vi "MNK_TC_to_DSC.vi"(8 "error in (no error)":errorcluster, 9 "calibration string":string, 10 "description string":string, 11 "dbl":dbl[](array[numeric])) -> (0 "error out":errorcluster)   [LabVIEW 2016]
panel:
  in  "calibration string var":refnum<k21>="ni.var.psp://housesoftheholy/MNK_18T/MNK_TC_calibration"
  in  "description string var":refnum<k21>="ni.var.psp://housesoftheholy/MNK_18T/MNK_TC_description"
  in  "dbl var":refnum<k21>[](array[refnum])=["ni.var.psp://housesoftheholy/MNK_18T/MNK_TC_R0", "ni.var.psp://housesoftheholy/MNK_18T/MNK_TC_R1", "ni.var.psp://housesoftheholy/MNK_18T/MNK_TC_R2", "ni.var.psp://housesoftheholy/MNK_18T/MNK_TC_R3", "ni.var.psp://housesoftheholy/MNK_18T/MNK_TC_R4", "ni.var.psp://housesoftheholy/MNK_18T/MNK_TC_R5", "ni.var.psp://housesoftheholy/MNK_18T/MNK_TC_R6", "ni.var.psp://housesoftheholy/MNK_18T/MNK_TC_R7", "ni.var.psp://housesoftheholy/MNK_18T/MNK_TC_T0", "ni.var.psp://housesoftheholy/MNK_18T/MNK_TC_T1", "ni.var.psp://housesoftheholy/MNK_18T/MNK_TC_T2", "ni.var.psp://housesoftheholy/MNK_18T/MNK_TC_T3", "ni.var.psp://housesoftheholy/MNK_18T/MNK_TC_T4", "ni.var.psp://housesoftheholy/MNK_18T/MNK_TC_T5", "ni.var.psp://housesoftheholy/MNK_18T/MNK_TC_T6", "ni.var.psp://housesoftheholy/MNK_18T/MNK_TC_T7", "ni.var.psp://housesoftheholy/MNK_18T/MNK_TC_I0", "ni.var.psp://housesoftheholy/MNK_18T/MNK_TC_I1", "ni.var.psp://housesoftheholy/MNK_18T/MNK_TC_I2", "ni.var.psp://housesoftheholy/MNK_18T/MNK_TC_I3", "", "", "", "", ""]
  # "MNK TC to DSC"
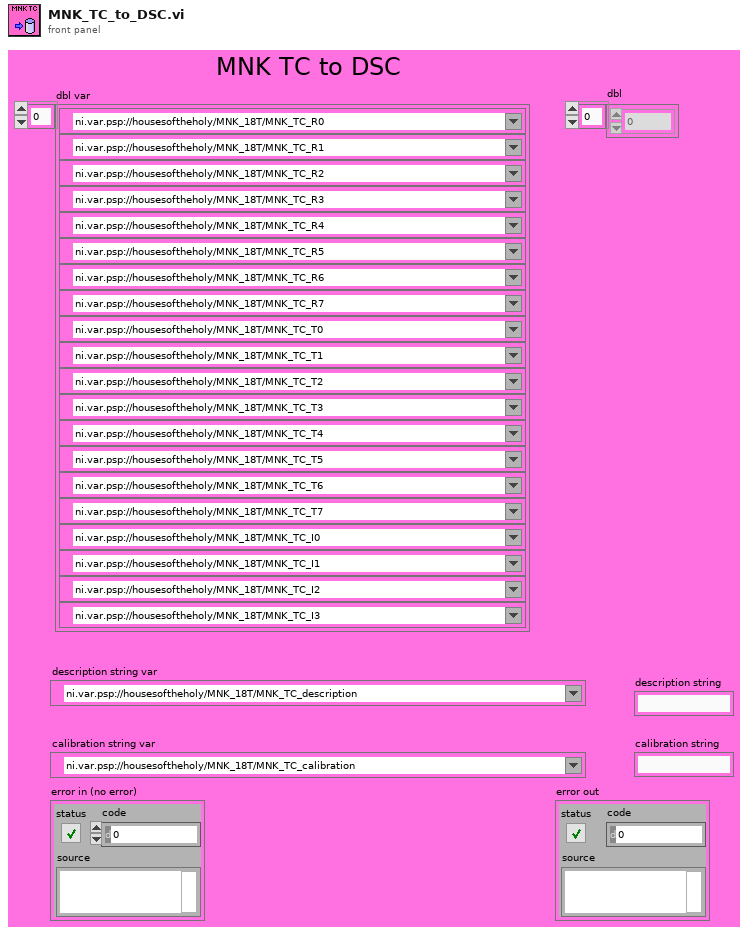
[diagram p1: front panel]
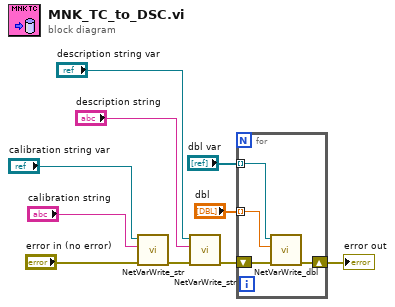
[diagram p0: block diagram]
diagram:
  n1 = call "NetVarWrite_str.vi"("error in (no error)"="error in (no error)", "String"="calibration string", "Refnum in"="calibration string var") -> ("error out"=w4:errorcluster)  [unwired: 8 in]
  n2 = call "NetVarWrite_str.vi"("error in (no error)"=w4, "String"="description string", "Refnum in"="description string var") -> ("error out"=w1:errorcluster)  [unwired: 8 in]
  n3 = for {
    tunnel: "dbl var" -> [w12] mode=indexing
    tunnel: "dbl" -> [w13] mode=indexing
    shift-right: [w11] -> w8
    shift-left: w1 -> [w14]
    n4 = call "NetVarWrite_dbl.vi"("error in (no error)"=w14, "Numeric"=w13, "Refnum in"=w12) -> ("error out"=w11:errorcluster)  [unwired: 8 in]
  }
  "error out" <- w8
